vi "FPGA_encoder_hall.vi"() -> ()   [LabVIEW 2019]
uses:
  <vilib>/rvi/Emulation/niFpgaGetClockAttributes.vi
  <vilib>/rvi/Emulation/niFpgaSctlEmulationGetInTimedLoop.vi
  <vilib>/rvi/Emulation/niFpgaEmulationReportErrorSimple.vi
  <vilib>/rvi/eio/common/nirviEmuTemplateMethod_errors.vi
  <vilib>/rvi/Emulation/niFpgaCriticalErrorInLSC.vi
  <vilib>/eio/EIONode/EIONode.xnode
panel:
  in  "Encoder Position Reset":bool
  out "Encoder (Counts)":i32
  out "ConnectorA/DIO0":bool
  out "Hall State":enum16{"Check Threshold", "Bounce Time"}(ring)
  out "Hall Period (uSec/pulse)":u32
  in  "Slope":enum16{"falling", "rising"}(ring)
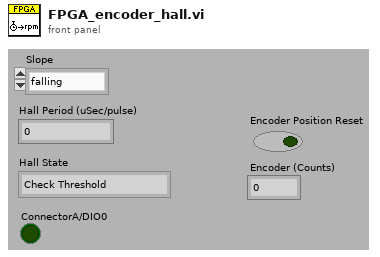
[diagram p1: front panel]
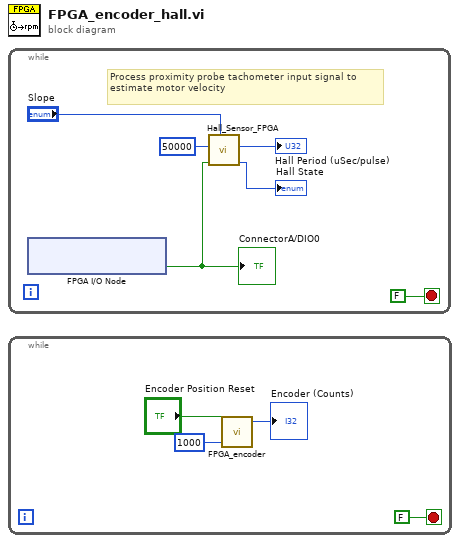
[diagram p0: block diagram]
diagram:
  n1 = while {
    stop <- FALSE stop-if-true
    # "Process proximity probe tachometer input signal to estimate motor velocity"
    n2 = xnode "FPGA I/O Node"() -> ("ConnectorA/DIO0"=w3:bool)  [unwired: 1 in, 1 out]
    "ConnectorA/DIO0" <- w3
    n3 = call "Hall_Sensor_FPGA.vi"("Slope"="Slope", "Hall Sensor"=w3, "Bounce time (uSec)"=u32 50000) -> ("State Out"=→"Hall State":enum16{"Check Threshold", "Bounce Time"}, "Tach Period (uSec/pulse)"=→"Hall Period (uSec/pulse)":u32)  [unwired: 7 in]
  }
  n4 = while {
    stop <- FALSE stop-if-true
    n5 = call "FPGA_encoder.vi"("Velocity Interval (uSec)"=u32 1000, "Position Reset"="Encoder Position Reset") -> ("Position (Counts)"=→"Encoder (Counts)":i32)  [unwired: 1 in, 2 out]
  }
